vi "ADO Type and Dir to DB Tools.vi"(4 "error in (no error)":errorcluster, 6 "ADO direction":u16(ring) items=["adParamUnknown", "adParamInput", "adParamOutput", "adParamInputOutput", "adParamReturnValue"], 7 "ADO type":i32(ring) items=["adEmpty"=0, "adTinyInt"=16, "adSmallInt"=2, "adInteger"=3, "adBigInt"=20, "adUnsignedTinyInt"=17, "adUnsignedSmallInt"=18, "adUnsignedInt"=19, "adUnsignedBigInt"=21, "adSingle"=4, "adDouble"=5, "adCurrency"=6, "adDecimal"=14, "adNumeric"=131, "adBoolean"=11, "adError"=10, "adUserDefined"=132, "adVariant"=12, "adIDispatch"=9, "adIUnknown"=13, "adGUID"=72, "adDate"=7, "adDBDate"=133, "adDBTime"=134, "adDBTimeStamp"=135, "adBSTR"=8, "adChar"=129, "adVarChar"=200, "adLongVarChar"=201, "adWChar"=130, "adVarWChar"=202, "adLongVarWChar"=203, "adBinary"=128, "adVarBinary"=204, "adLongVarBinary"=205, "adChapter"=136, "adFileTime"=64, "adDBFileTime"=137, "adPropVariant"=138, "adVarNumeric"=139]) -> (0 "error out":errorcluster, 2 "direction":T2, 3 "data type":T1)   [LabVIEW 2013, in "NI_Database_API_64.lvlib"]
doc: "Converts the ADO data type and parameter direction to the values used by the database tools."
uses:
  NI_Database_API_64.lvlib
  DB Tools Parameter Dir.ctl
  DB Tools DataTypes.ctl
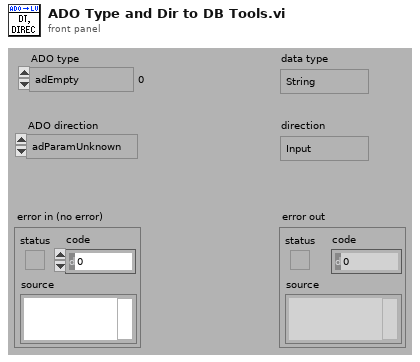
[diagram p1: front panel]
types:
  T1 = typedef "NI_Database_API_64.lvlib/DB Tools DataTypes.ctl" = enum16{"String", "Long (I32)", "Single (SGL)", "Double (DBL)", "Date/Time", "Binary"}
  T2 = typedef "NI_Database_API_64.lvlib/DB Tools Parameter Dir.ctl" = enum32{"Input", "Output", "Input/Output", "Return Value"}
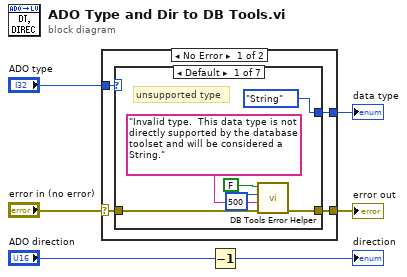
[diagram p0: block diagram]
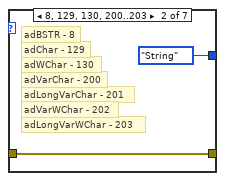
[diagram p2: hidden frame]
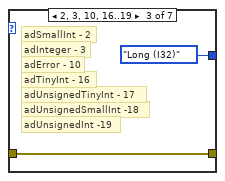
[diagram p3: hidden frame]
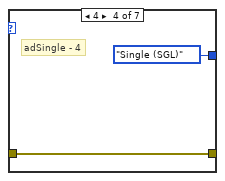
[diagram p4: hidden frame]
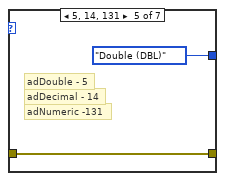
[diagram p5: hidden frame]
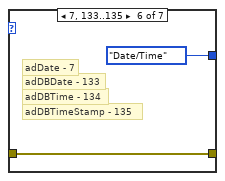
[diagram p6: hidden frame]
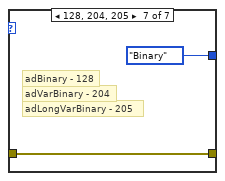
[diagram p7: hidden frame]
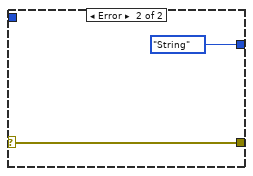
[diagram p8: hidden frame]
diagram:
  n1 = case shown="No Error" "error in (no error)" {
    selector: "error in (no error)" -> [w7 w30]
    tunnel: "ADO type" -> [w10 _]
    tunnel: [w9 DB_Tools_DataTypes."String" ("Data Type")] -> w2
    tunnel: [w8 w30] -> w1
    frame No Error {
      n2 = case shown="Default" w10 {
        tunnel: [DB_Tools_DataTypes."String" ("Data Type") DB_Tools_DataTypes."String" ("Data Type") DB_Tools_DataTypes."Long (I32)" ("Data Type") DB_Tools_DataTypes."Single (SGL)" ("Data Type") DB_Tools_DataTypes."Double (DBL)" ("Data Type") DB_Tools_DataTypes."Date/Time" ("Data Type") DB_Tools_DataTypes."Binary" ("Data Type")] -> w9
        tunnel: w7 -> [w11 w17 w19 w21 w23 w25 w27]
        tunnel: [w15 w17 w19 w21 w23 w25 w27] -> w8
        frame Default {
          # "unsupported type"
          n3 = call "DB Tools Error Helper.vi"("Overriding error or warning"=w11, "source"="Invalid type.  This data type is not directly supported by the database toolset and will be considered a String.", "code"=500, "status"=FALSE) -> ("error out"=w15:errorcluster)  [unwired: 7 out]
        }
        frame 8, 129, 130, 200..203 {
          # "adChar - 129"
          # "adWChar - 130"
          # "adBSTR - 8"
          # "adLongVarWChar - 203"
          # "adVarWChar - 202"
          # "adLongVarChar - 201"
          # "adVarChar - 200"
        }
        frame 2, 3, 10, 16..19 {
          # "adUnsignedInt -19"
          # "adSmallInt - 2"
          # "adUnsignedSmallInt -18"
          # "adUnsignedTinyInt - 17"
          # "adTinyInt - 16"
          # "adError - 10"
          # "adInteger - 3"
        }
        frame 4 {
          # "adSingle - 4"
        }
        frame 5, 14, 131 {
          # "adDouble - 5"
          # "adDecimal - 14"
          # "adNumeric -131"
        }
        frame 7, 133..135 {
          # "adDate - 7"
          # "adDBTime - 134"
          # "adDBDate - 133"
          # "adDBTimeStamp - 135"
        }
        frame 128, 204, 205 {
          # "adBinary - 128"
          # "adLongVarBinary - 205"
          # "adVarBinary - 204"
        }
      }
    }
    frame Error {
    }
  }
  "data type" <- w2
  "error out" <- w1
  n4 = Decrement(x="ADO direction") -> (x-1=→"direction":u16)
